vi "AprilTag Interpolator.vi"(8 "Current Angle (deg)":dbl=141.0 format="%0.2f", 11 "Interpolation Table":dbl[][](array[numeric])=[[-68.0, -44.0, -32.0, 12.0, 46.0, 74.0], [-23.0, -8.0, -4.2, 5.6, 11.0, 19.0]] format="%0.2f") -> (3 "Corrected Angle (deg)":dbl=133.0 format="%0.2f")   [LabVIEW 2023]
uses:
  <vilib>/Analysis/NI_AALPro.lvlib
panel:
  # "We train these values when we set up the shooter. We can also add these to the dashboard so we can tweak them. This will make setting up our shooter simple and easy to adjust."
  # "We output this number to the PID loop to control the speed of the shooter."
  # "We get the distance from the vision software and feed it into the interpolator."
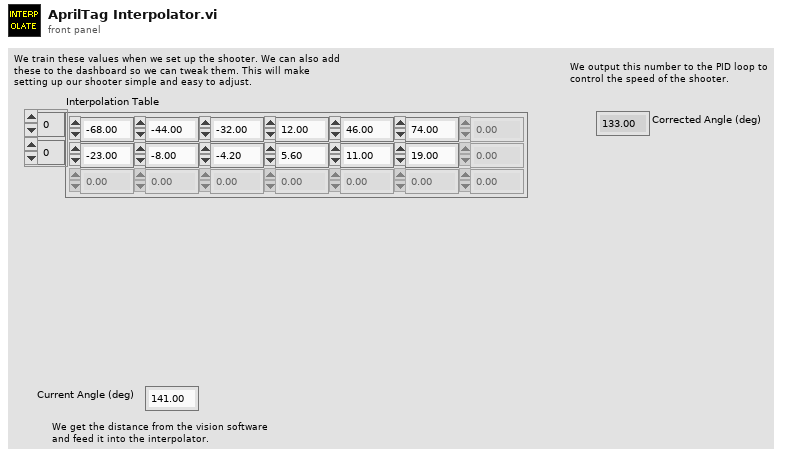
[diagram p1: front panel]
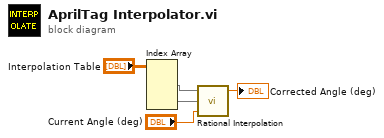
[diagram p0: block diagram]
diagram:
  n1 = Index Array(array="Interpolation Table") -> (element #1=w4:dbl[], element #2=w3:dbl[])  [unwired: 4 in]
  n2 = call <vilib>:"Rational Interpolation.vi"("x value"="Current Angle (deg)", "X"=w3, "Y"=w4) -> ("interpolation value"=→"Corrected Angle (deg)":dbl)  [unwired: 2 out]
